vi "SubPanel_UI.vi"(0 "Front Panel":refnum<vi>, 1 "Panel Bounds":T2, 2 "SubNumber":i32=8, 3 "SubPanelRows":i32=2, 4 "ItemSize":i32=2, 5 "error in":errorcluster, 6 "Mark_Position":T1) -> (14 "SubPanarray":refnum<vi>[](array[refnum]), 19 "error out":errorcluster)   [LabVIEW 2014]
uses:
  <vilib>/Utility/miscctls.llb/LVPositionTypeDef.ctl
  <vilib>/Utility/miscctls.llb/LVRectTypeDef.ctl
panel:
  in  "Position":T1
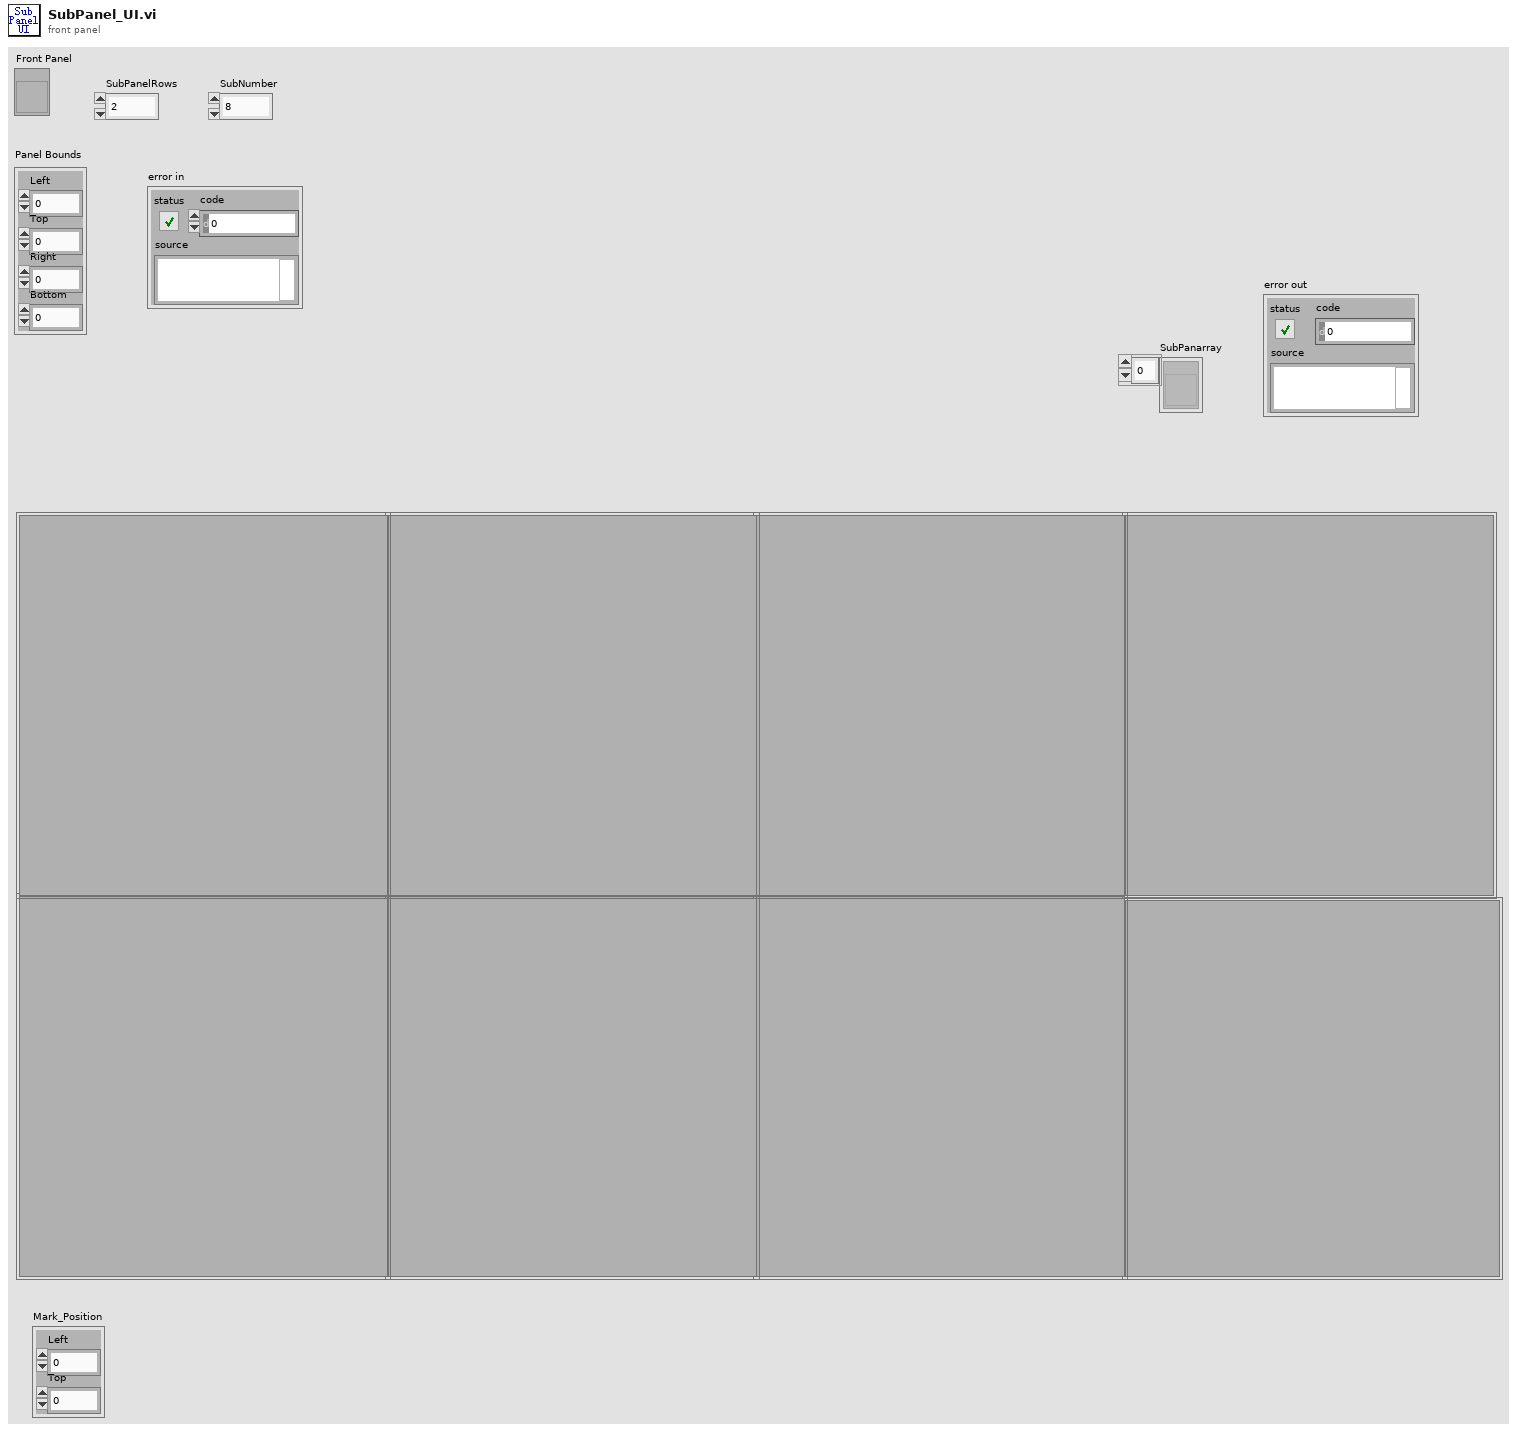
[diagram p1: front panel]
types:
  T1 = typedef "LVPositionTypeDef.ctl" = cluster{"Left":i32, "Top":i32}
  T2 = typedef "LVRectTypeDef.ctl" = cluster{"Left":i16, "Top":i16, "Right":i16, "Bottom":i16}
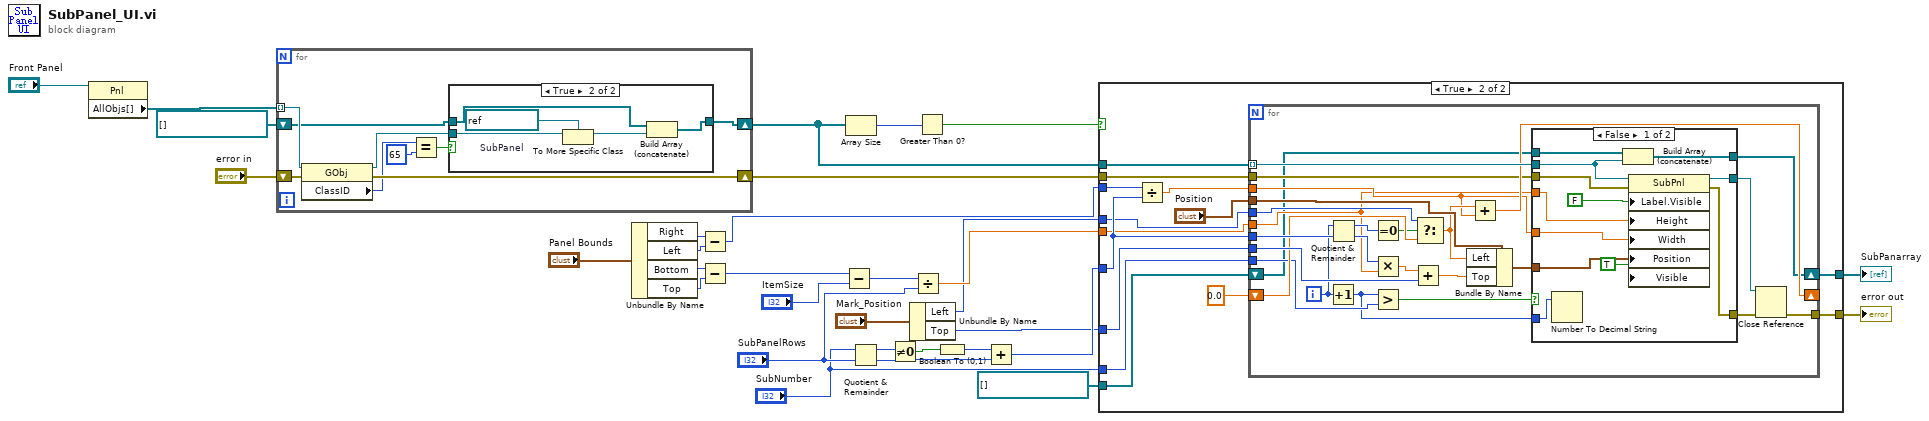
[diagram p0: block diagram]
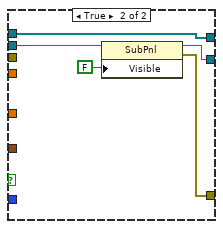
[diagram p3: hidden frame]
diagram:
  n1 = property class="Pnl"(reference="Front Panel") -> ("AllObjs[]"=w28:refnum<vi>[])  [unwired: 1 in, 2 out]
  n2 = for {
    tunnel: w28 -> [w40] mode=indexing
    shift-right: [w35] -> w15
    shift-left: refnum<vi>[] [] -> [w34]
    shift-right: [w33] -> w18
    shift-left: "error in" -> [w39]
    n3 = property class="GObj"(reference=w40, error in=w39) -> (reference out=w36:refnum<vi>, error out=w33:errorcluster, "ClassID"=w32:u32)
    n4 = Equal?(x=w32, y=u32 65) -> (x = y?=w37:bool)
    n5 = case shown="True" w37 {
      tunnel: w36 -> [_ w46]
      tunnel: [w41 w43] -> w35
      tunnel: w34 -> [w41 w42]
      frame False {
      }
      frame True {
        w45 = refnum<vi> refnum  # SubPanel
        n6 = To More Specific Class(target class=w45, reference=w46) -> (specific class reference=w44:refnum<vi>)  [unwired: 1 in, 1 out]
        n7 = Build Array (concatenate)(w42, w44) -> (w43:refnum<vi>[])
      }
    }
  }
  n8 = Unbundle By Name("Panel Bounds") -> ("Right"=w31:i16, "Left"=w21:i16, "Bottom"=w30:i16, "Top"=w22:i16)
  n9 = Subtract(x=w31, y=w21) -> (x-y=w19:i16)
  n10 = Subtract(x=w30, y=w22) -> (x-y=w9:i16)
  n11 = Subtract(x=w9, y="ItemSize") -> (x-y=w8:i32)
  n12 = Array Size(array=w15) -> (size(s)=w26:i32)
  n13 = Quotient & Remainder(x="SubNumber", y="SubPanelRows") -> (x-y*floor(x/y)=w2:i32, floor(x/y)=w24:i32)
  n14 = Not Equal To 0?(x=w2) -> (x != 0?=w3:bool)
  n15 = Unbundle By Name("Mark_Position") -> ("Left"=w5:i32, "Top"=w4:i32)
  n16 = Divide(x=w8, y="SubPanelRows") -> (x/y=w25:dbl)
  n17 = Greater Than 0?(x=w26) -> (x > 0?=w27:bool)
  n18 = Boolean To (0,1)(Boolean=w3) -> (0, 1=w1:i16)
  n19 = Add(x=w1, y=w24) -> (x+y=w23:i32)
  n20 = case shown="True" w27 {
    tunnel: w15 -> [_ w62]
    tunnel: w25 -> [_ w50]
    tunnel: w19 -> [_ w61]
    tunnel: w23 -> [_ w56]
    tunnel: w4 -> [_ w49]
    tunnel: w5 -> [_ w51]
    tunnel: "SubNumber" -> [_ w57]
    tunnel: w18 -> [w48 w55]
    tunnel: [w48 w54] -> w17
    tunnel: [w47 w53] -> w13
    tunnel: refnum<vi>[] [] ("SubPanarray") -> [w47 w52]
    frame False {
    }
    frame True {
      n21 = Divide(x=w61, y=w56) -> (x/y=w60:dbl)
      n22 = for {
        tunnel: w62 -> [w88] mode=indexing
        tunnel: "Position" -> [w87]
        tunnel: w51 -> [w77]
        tunnel: w60 -> [w68]
        tunnel: w50 -> [w67]
        tunnel: w49 -> [w80]
        tunnel: w56 -> [w81]
        shift-right: [w82] -> _
        shift-left: 0.0 ("y") -> [w78]
        tunnel: w57 -> [w76]
        tunnel: w55 -> [w66]
        tunnel: [w65] -> w54
        shift-right: [w63] -> w53
        shift-left: w52 -> [w64]
        i -> [w75]
        n23 = Increment(x=w75) -> (x+1=w71:i32)
        n24 = Quotient & Remainder(x=w75, y=w81) -> (x-y*floor(x/y)=w74:i32, floor(x/y)=w72:i32)
        n25 = Equal To 0?(x=w74) -> (x = 0?=w73:bool)
        n26 = Multiply(x=w72, y=w67) -> (x*y=w79:dbl)
        n27 = Greater?(x=w71, y=w76) -> (0:w85:bool)
        n28 = Add(x=w79, y=w80) -> (x+y=w69:dbl)
        n29 = Select(t=w77, s=w73, f=w78) -> (s? t:f=w70:dbl)
        n30 = Bundle By Name(cluster=w87, "Left"=w70, "Top"=w69) -> (w86:T1)
        n31 = Add(x=w70, y=w68) -> (x+y=w82:dbl)
        n32 = case shown="False" w85 {
          tunnel: w88 -> [w90 w105]
          tunnel: w86 -> [w100 _]
          tunnel: w67 -> [w94 _]
          tunnel: w68 -> [w93 _]
          tunnel: [w99 w103] -> w84
          tunnel: [w98 w104] -> w83
          tunnel: w71 -> [w97 _]
          tunnel: w66 -> [w92 _]
          tunnel: w64 -> [w91 w101]
          tunnel: [w89 w101] -> w63
          frame False {
            n33 = Number To Decimal String(number=w97) -> ()  [unwired: 1 in, 1 out]
            n34 = Build Array (concatenate)(w91, w90) -> (w89:refnum<vi>[])
            n35 = property class="SubPnl"(reference=w90, error in=w92, "Label.Visible"=FALSE, "Height"=w94, "Width"=w93, "Position"=w100, "Visible"=TRUE) -> (reference out=w98:refnum<vi>, error out=w99:errorcluster)
          }
          frame True {
            n36 = property class="SubPnl"(reference=w105, "Visible"=FALSE) -> (reference out=w104:refnum<vi>, error out=w103:errorcluster)  [unwired: 1 in]
          }
        }
        n37 = Close Reference(reference=w83, error in (no error)=w84) -> (error out=w65:errorcluster)
      }
    }
  }
  "error out" <- w17
  "SubPanarray" <- w13
